vi "Initialize.vi"(8 "error in (no error)":errorcluster, 11 "Qbus":refnum<class "Qbus.lvclass">) -> (0 "error out":errorcluster, 3 "config":T1)   [LabVIEW 2017, in "McsaModbusMaster.lvlib"]
uses:
  <vilib>/addons/InsightCM/Devices/Shared/Mcsa/McsaModbusMaster/McsaModbusMaster.lvlib
  <vilib>/addons/InsightCM/Devices/Shared/Common/ModbusMaster/controls/config.ctl
  <vilib>/addons/InsightCM/Devices/Shared/Common/ModbusMaster/controls/ModbusDevice.ctl
  <vilib>/Modbus/master/Modbus Master.lvclass
  <vilib>/addons/InsightCM/Devices/Shared/Common/ModbusMaster/controls/ModbusChannel.ctl
  <vilib>/addons/InsightCM/Devices/Shared/Common/ModbusMaster/controls/RegisterType.ctl
  <vilib>/addons/InsightCM/MessageBus/Base/controls/DataSource.ctl
  <vilib>/addons/InsightCM/MessageBus/Base/controls/KeyValuePair.ctl
  <vilib>/addons/Qbus/Qbus.lvclass
  <vilib>/addons/InsightCM/Devices/Shared/Common/ModbusMaster/ModbusMaster.lvlib
  <vilib>/addons/InsightCM/Devices/Shared/Common/DataEventCreator/DataEventCreator.lvlib
  <vilib>/addons/InsightCM/Devices/Shared/Mcsa/McsaDataEventCreator/McsaDataEventCreator.lvlib
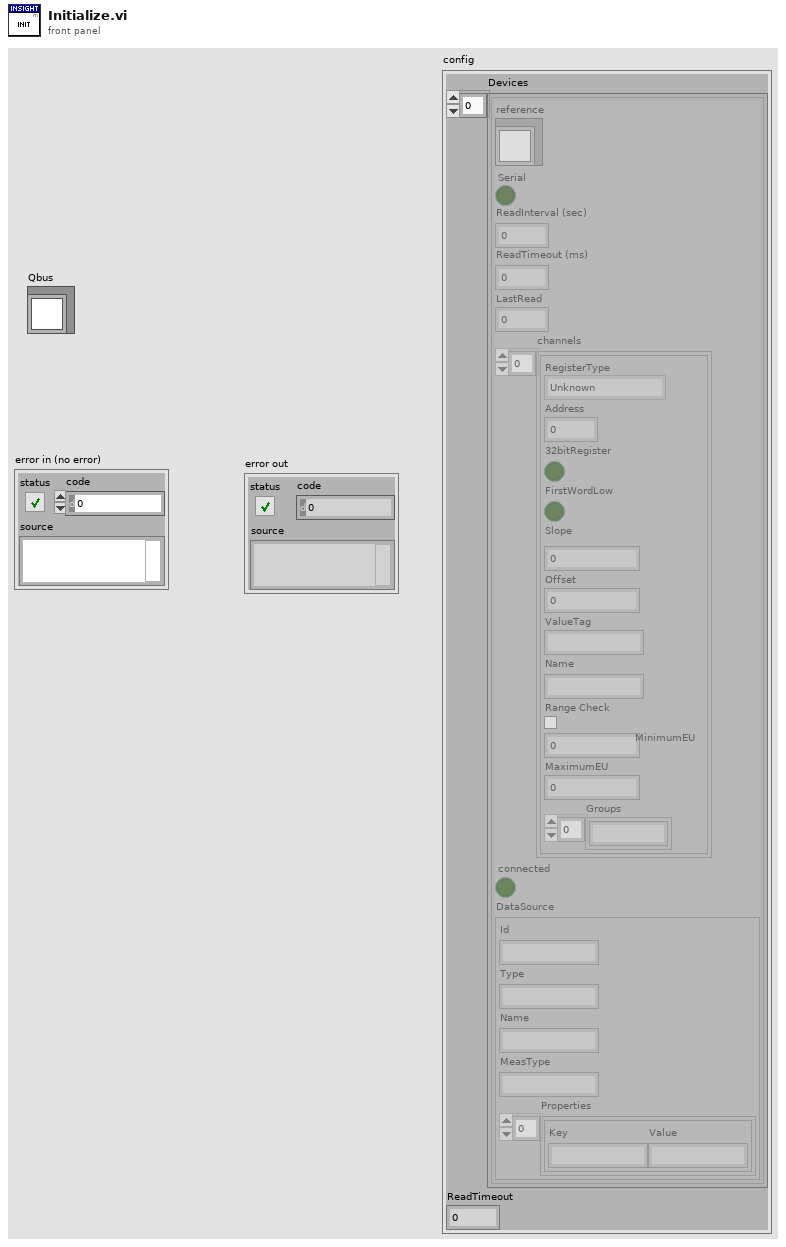
[diagram p1: front panel]
types:
  T1 = typedef "ModbusMaster.lvlib/config.ctl" = cluster{"Devices":T2[], "ReadTimeout":i32}
  T2 = typedef "ModbusMaster.lvlib/ModbusDevice.ctl" = cluster{"reference":refnum<class "Modbus Master.lvclass">, "Serial":bool, "ReadInterval (sec)":dbl, "ReadTimeout (ms)":i32, "LastRead":dbl, "channels":T3[], "connected":bool, "DataSource":T5}
  T3 = typedef "ModbusMaster.lvlib/ModbusChannel.ctl" = cluster{"RegisterType":T4, "Address":i32, "32bitRegister":bool, "FirstWordLow":bool, "Slope":dbl, "Offset":dbl, "ValueTag":string, "Name":string, "Range Check":bool, "MinimumEU":dbl, "MaximumEU":dbl, "Groups":string[]}
  T4 = typedef "ModbusMaster.lvlib/RegisterType.ctl" = enum16{"Unknown", "Coil", "Discrete Input", "Holding Register", "Input Register"}
  T5 = typedef "DataSource.ctl" = cluster{"Id":string, "Type":string, "Name":string, "MeasType":string, "Properties":T6[]}
  T6 = typedef "KeyValuePair.ctl" = cluster{"Key":string, "Value":string}
  T7 = typedef "DataEventCreator.lvlib/RegisterTrendPoints.ctl" = cluster{"DataGroup":string, "Trends":T8[]}
  T8 = typedef "DataEventCreator.lvlib/Registry_Trend.ctl" = cluster{"TrendPointId":string, "DataSetName":string, "HighRate":bool, "Always Send":bool}
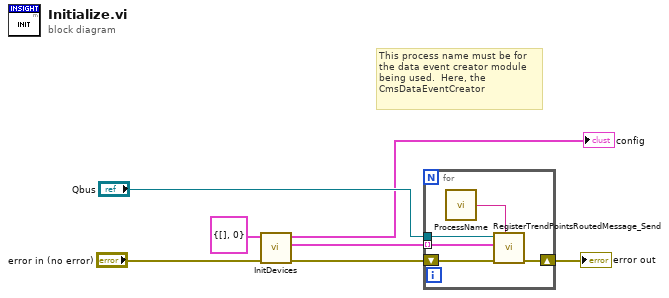
[diagram p0: block diagram]
diagram:
  # "This process name must be for\nthe data event creator module\nbeing used.  Here, the \nCmsDataEventCreator"
  n1 = call <vilib>:"InitDevices.vi"("error in (no error)"="error in (no error)", "config in"=T1 {"Devices"=[], "ReadTimeout"=0} ("config")) -> ("error out"=w2:errorcluster, "register trends"=w1:T7[], "config out"=→"config":T1)  [unwired: 7 in]
  n2 = for {
    tunnel: w1 -> [w10] mode=indexing
    shift-right: [w11] -> w7
    shift-left: w2 -> [w12]
    tunnel: "Qbus" -> [w9]
    n3 = call <vilib>:"ProcessName.vi"() -> ("process name"=w8:string)  [unwired: 5 in]
    n4 = call <vilib>:"RegisterTrendPointsRoutedMessage_Send.vi"("data event creator process name"=w8, "error in (no error)"=w12, "register trend"=w10, "Qbus in"=w9) -> ("error out"=w11:errorcluster)  [unwired: 6 in, 1 out]
  }
  "error out" <- w7
